vi "Write Hyperdrive class.vi"(8 "error in (no error)":errorcluster, 10 "Hyperdrive class":T1(ring), 11 "Hyperspace_SpaceShip in":refnum<class "Hyperspace_SpaceShip.lvclass">) -> (0 "error out":errorcluster, 3 "Hyperspace_SpaceShip out":refnum<class "Hyperspace_SpaceShip.lvclass">)   [LabVIEW 2021, in "Hyperspace_SpaceShip.lvclass"]
uses:
  Hyperspace_SpaceShip.lvclass
  Hyperspace_SpaceShip.lvclass/Hyperspace_SpaceShip.ctl
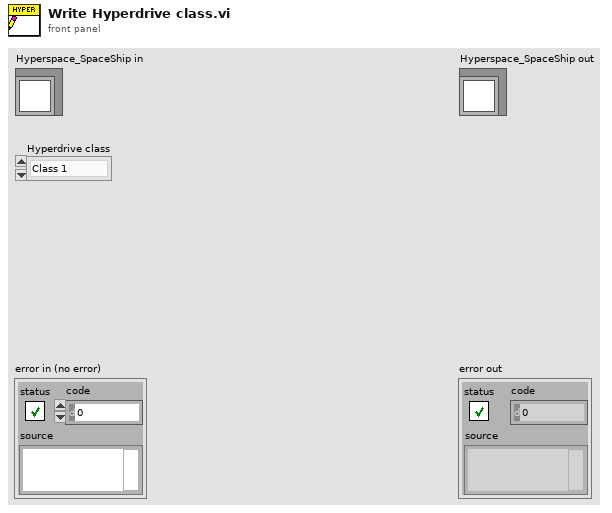
[diagram p1: front panel]
types:
  T1 = enum16{"Class 1", "Class 2", "Class 3", "Class 4"}
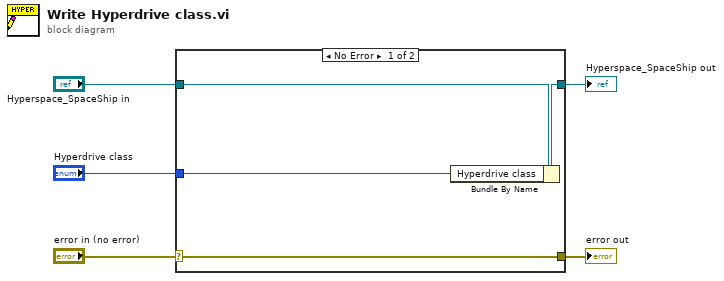
[diagram p0: block diagram]
diagram:
  n1 = case shown="No Error" "error in (no error)" {
    selector: "error in (no error)" -> [w9 w10]
    tunnel: [w9 w10] -> w4
    tunnel: [w7 w11] -> w2
    tunnel: "Hyperspace_SpaceShip in" -> [w8 w11]
    tunnel: "Hyperdrive class" -> [w6 _]
    frame No Error {
      n2 = Bundle By Name(cluster=w8, "Hyperdrive class"=w6) -> (w7:refnum<class "Hyperspace_SpaceShip.lvclass">)
    }
    frame Error {
    }
  }
  "error out" <- w4
  "Hyperspace_SpaceShip out" <- w2
